vi "find best direction.vi"(9 "Objects":T1[](array[typedef]), 11 "current location":cluster{"x":i16, "y":i16}) -> (1 "magnitude":sgl(slide) scale=-10.0..10.0, 3 "Direction":sgl(knob) scale=-3.14..3.14)   [LabVIEW 2009]
uses:
  object.ctl
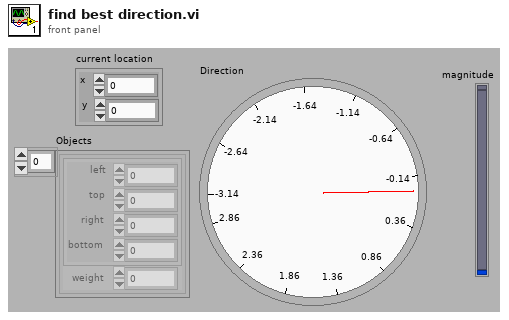
[diagram p1: front panel]
types:
  T1 = typedef "object.ctl" = cluster{"rect":cluster{"left":i16, "top":i16, "right":i16, "bottom":i16}, "weight":sgl}
  T2 = typedef "object relations.ctl" = cluster{"closest point":cluster{"x":i16, "y":i16}, "theta":sgl, "intersect angle":sgl, "distance":i16, "area":i16, "weight":sgl, "d from center":i16}
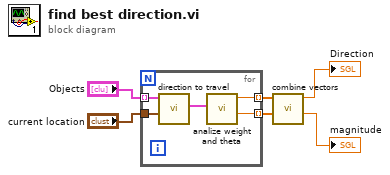
[diagram p0: block diagram]
diagram:
  n1 = for {
    tunnel: "current location" -> [w11]
    tunnel: "Objects" -> [w10] mode=indexing
    tunnel: [w9] -> w3 mode=indexing
    tunnel: [w8] -> w4 mode=indexing
    n2 = call "direction to travel.vi"("current location"=w11, "rectangle object"=w10) -> ("relative object data"=w7:T2)  [unwired: 9 in]
    n3 = call "analize weight and theta.vi"("relative object data"=w7) -> ("weight"=w8:sgl, "theta"=w9:sgl)  [unwired: 9 in]
  }
  n4 = call "combine vectors.vi"("magnitudes"=w4, "directions"=w3) -> ("magnitude"=→"magnitude":sgl, "direction"=→"Direction":sgl)  [unwired: 8 in]
